vi "get device CstrSerialNumber.vi"() -> ()   [LabVIEW 2013, in "libusvlv.lvlib"]
uses:
  libusvlv.lvlib
  UsbCom.dll
panel:
  in  "byte buffer":string
  out "len":i32
  out "SerialNumber":string
  in  "len":i32
  in  "index":i32
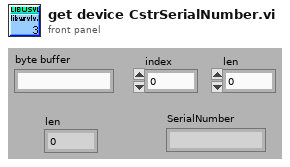
[diagram p1: front panel]
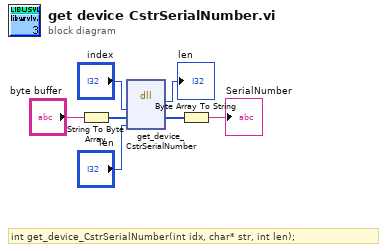
[diagram p0: block diagram]
diagram:
  # "int get_device_CstrSerialNumber(int idx, char* str, int len);"
  n1 = String To Byte Array(string="byte buffer") -> (unsigned byte array=w1:u8[])
  n2 = dll-call lib="E:/libusvlv/UsbCom.dll" fn="get_device_CstrSerialNumber"("idx"="index", "str"=w1, "len"="len") -> ("size"=→"len":i32, "str"=w5:i8[])  [unwired: 5 in, 2 out]
  n3 = Byte Array To String(unsigned byte array=w5) -> (string=→"SerialNumber":string)
